vi "Update.vi"(8 "error in (no error)":errorcluster, 11 "Motions in":refnum<class "Motions.lvclass">) -> (0 "error out":errorcluster, 3 "Motions out":refnum<class "Motions.lvclass">)   [LabVIEW 2016, in "Hardware.lvlib" / "Motions.lvlib" / "Motions.lvclass"]
uses:
  <userlib>/Common Components/Hardware/Abstract System/Motions/Motions/Motions.lvclass
  <userlib>/Common Components/Hardware/Abstract System/Motions/Motions/Motions.lvclass/Motions.ctl
  <userlib>/Common Components/TriggerAction Q/TriggerAction Q/TriggerAction Q.lvclass/TriggerAction Q.ctl
  <userlib>/Common Components/TriggerAction Q/TriggerAction Q/Run (non-indexed).vi
  <userlib>/Common Components/Hardware/Motor/Motor/Motor.lvclass
  <userlib>/Common Components/TriggerAction Q/TriggerAction Q/TriggerAction Q.lvclass
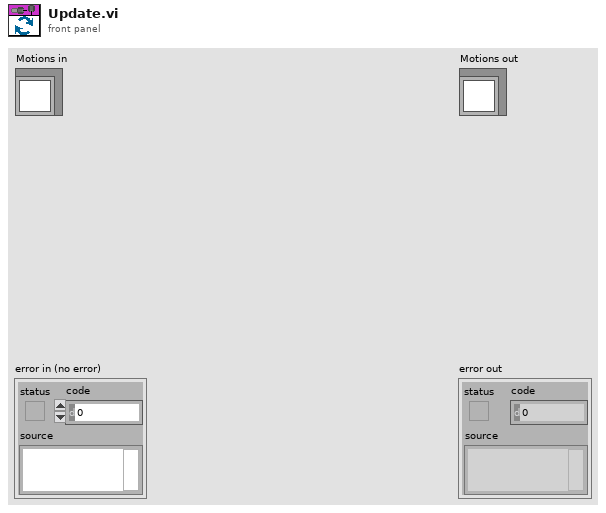
[diagram p1: front panel]
types:
  T1 = typedef "Hardware.lvlib/Motions.lvlib/Motions.lvclass/Motor States.ctl" = cluster{"Connected":bool, "Enabled":bool, "Moving Status":bool, "Soft Moving Status":bool, "Current Pos":dbl, "Target Pos":dbl, "Moving Dir (-1, 0, 1)":i32, "Error Status":bool, "Hard Limit+":bool, "Hard Limit-":bool, "Soft Limit+":bool, "Soft Limit-":bool, "History Dst Stack":refnum<queue>, "Motion Status":bool, "Motion TriggerAction Obj":refnum<class "TriggerAction Q.lvclass">, "Jogging":bool}
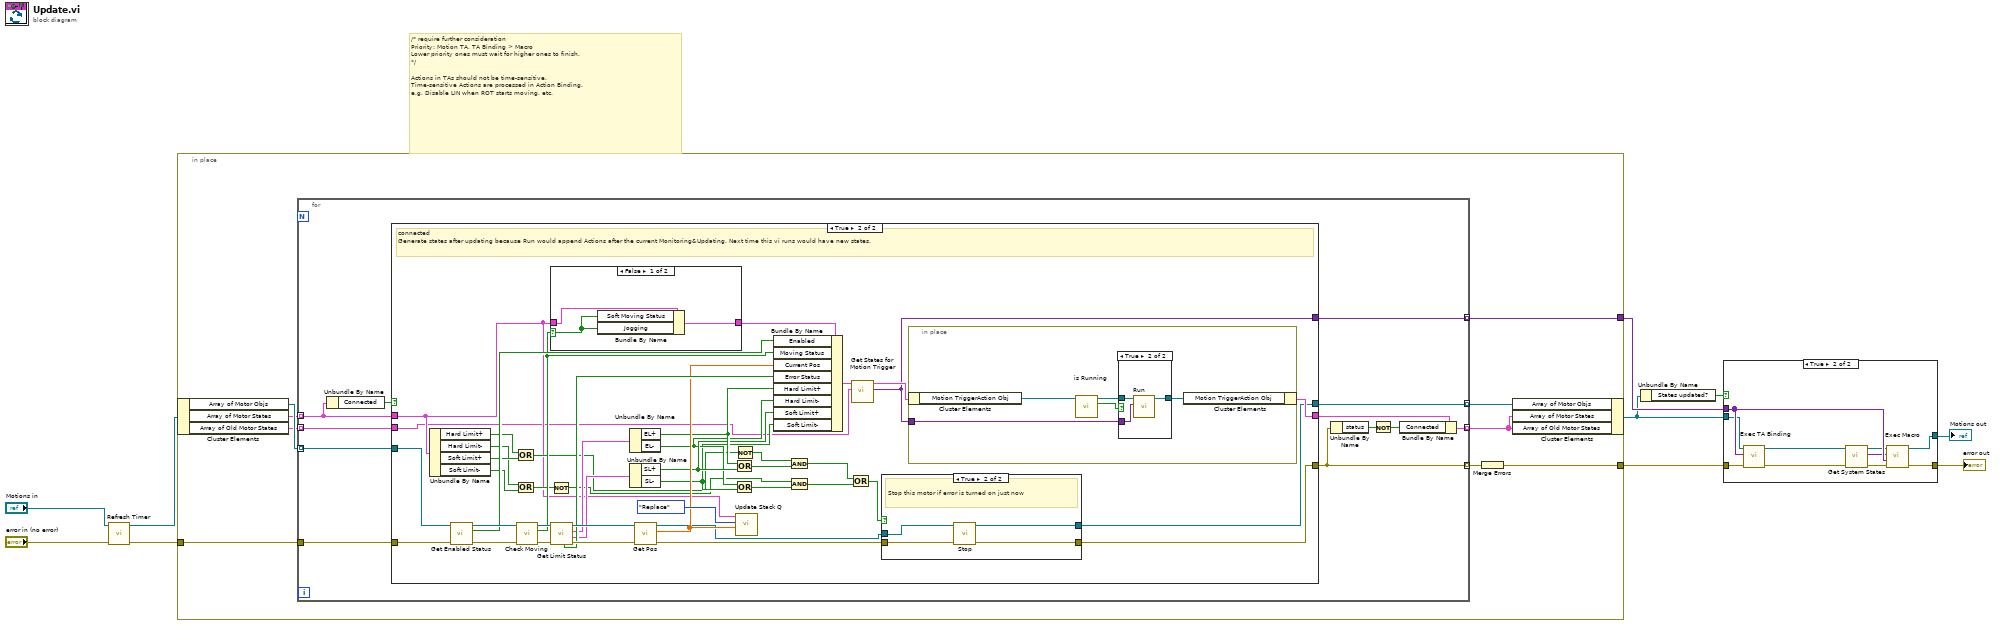
[diagram p0: block diagram]
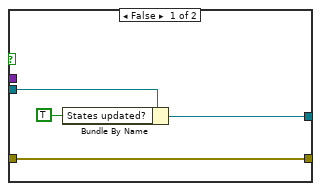
[diagram p2: hidden frame]
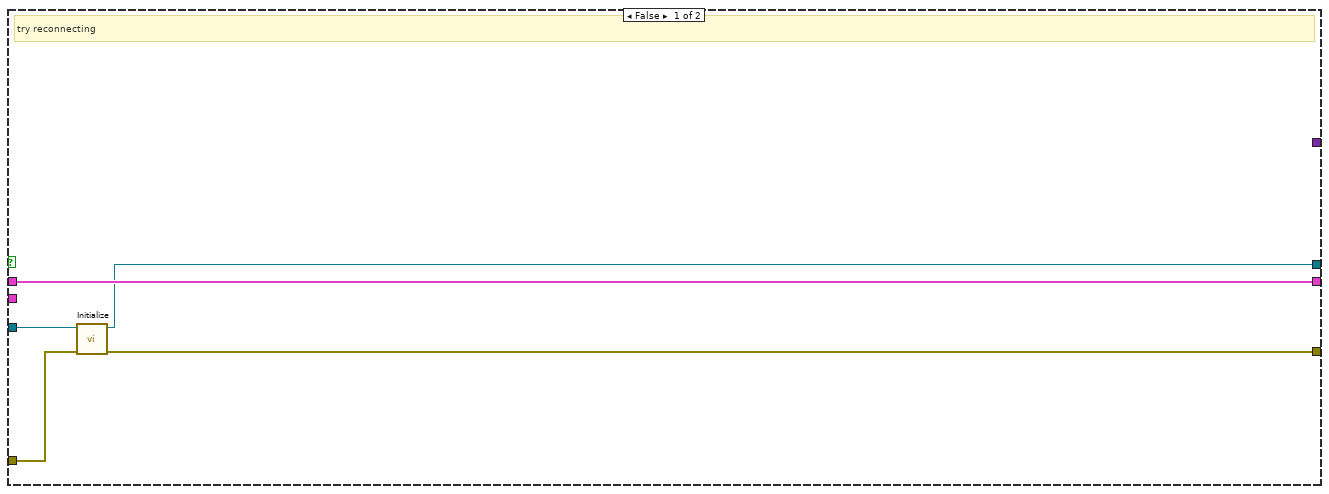
[diagram p3: hidden frame]
diagram:
  # "/* require further consideration\nPriority: Motion TA, TA Binding > Macro\nLower priority ones must wait for higher ones to finish.\n*/\n\nActions in TAs should not be time-sensitive.\nTime-sensitive Actions are processed in Action Binding.\ne.g. Disable LIN when ROT starts moving, etc."
  n1 = call <userlib>:"Refresh Timer.vi"("error in (no error)"="error in (no error)", "Motions in"="Motions in") -> ("error out"=w6:errorcluster, "Motions out"=w4:refnum<class "Motions.lvclass">)  [unwired: 8 in]
  n2 = in-place {
    in-place-border: w6 -> [w19]
    in-place-border: [w17] -> w9
    in-place-border: [w13] -> w3
    n3 = in-place-cluster #1(w4) -> ("Array of Motor Objs"=w16:refnum<class "Motor.lvclass">[], "Array of Motor States"=w15:T1[], "Array of Old Motor States"=w12:T1[])
    n4 = for {
      tunnel: w16 -> [w31] mode=indexing
      tunnel: w15 -> [w30] mode=indexing
      tunnel: [w26] -> w11 mode=indexing
      tunnel: w19 -> [w27]
      tunnel: [w25] -> w18 mode=indexing
      tunnel: [w22] -> w14 mode=indexing
      tunnel: [w21] -> w13 mode=indexing
      tunnel: w12 -> [w20] mode=indexing
      n5 = Unbundle By Name(w30) -> ("Connected"=w29:bool)
      n6 = case shown="True" w29 {
        tunnel: w31 -> [w35 w79]
        tunnel: w30 -> [w36 w38]
        tunnel: [w36 w63] -> w28
        tunnel: w27 -> [w34 w75]
        tunnel: [w33 w42] -> w25
        tunnel: [w32 w40] -> w22
        tunnel: [_ w59] -> w21
        tunnel: w20 -> [_ w37]
        frame False {
          # "try reconnecting"
          n7 = call-dynamic "Initialize.vi"("error in (no error)"=w34, "CCD in"=w35) -> ("error out"=w33:errorcluster, "CCD out"=w32:refnum<class "Motor.lvclass">)  [unwired: 8 in]
        }
        frame True {
          # "connected\nGenerate states after updating because Run would append Actions after the current Monitoring&Updating. Next time this vi runs would have new states."
          n8 = Unbundle By Name(w38) -> ("Hard Limit+"=w58:bool, "Hard Limit-"=w55:bool, "Soft Limit+"=w56:bool, "Soft Limit-"=w57:bool)
          n9 = call-dynamic "Get Enabled Status.vi"("error in (no error)"=w75, "Motor in"=w79) -> ("error out"=w74:errorcluster, "bENA"=w77:bool, "Motor out"=w78:refnum<class "Motor.lvclass">)  [unwired: 7 in]
          n10 = Or(x=w58, y=w56) -> (x .or. y?=w50:bool)
          n11 = Or(x=w55, y=w57) -> (x .or. y?=w47:bool)
          n12 = call-dynamic "Check Moving.vi"("error in (no error)"=w74, "Motor in"=w78) -> ("error out"=w73:errorcluster, "moving?"=w62:bool, "Motor out"=w70:refnum<class "Motor.lvclass">)  [unwired: 7 in]
          n13 = Not(x=w47) -> (.not. x?=w45:bool)
          n14 = case shown="False" w62 {
            selector: w62 -> [w95 _]
            tunnel: w38 -> [w97 w98]
            tunnel: [w96 w98] -> w76
            frame False {
              n15 = Bundle By Name(cluster=w97, "Soft Moving Status"=w95, "Jogging"=w95) -> (w96:T1)
            }
            frame True {
            }
          }
          n16 = call-dynamic "Get Limit Status.vi"("error in (no error)"=w73, "Motor in"=w70) -> ("error out"=w71:errorcluster, "Soft Limit status"=w66:cluster{"SL+":bool, "SL-":bool}, "EL status"=w67:cluster{"EL+":bool, "EL-":bool}, "Motor out"=w69:refnum<class "Motor.lvclass">, "ensemble Limit status"=w68:bool)  [unwired: 5 in]
          n17 = Unbundle By Name(w67) -> ("EL+"=w54:bool, "EL-"=w52:bool)
          n18 = Unbundle By Name(w66) -> ("SL+"=w53:bool, "SL-"=w51:bool)
          n19 = call <userlib>:"Get Pos.vi"("error in (no error)"=w71, "Motor in"=w69) -> ("error out"=w72:errorcluster, "Position in display unit (backend)"=w60:dbl, "Motor out"=w41:refnum<class "Motor.lvclass">)  [unwired: 6 in, 1 out]
          n20 = Or(x=w54, y=w53) -> (x .or. y?=w49:bool)
          n21 = Or(x=w52, y=w51) -> (x .or. y?=w46:bool)
          n22 = Not(x=w50) -> (.not. x?=w48:bool)
          n23 = call <userlib>:"Update Stack Q.vi"("Destination"=w60, "Mode"=enum16{"Add", "Replace"}."Replace", "Motor States"=w38) -> ()  [unwired: 9 in]
          n24 = Bundle By Name(cluster=w76, "Enabled"=w77, "Moving Status"=w62, "Current Pos"=w60, "Error Status"=w68, "Hard Limit+"=w54, "Hard Limit-"=w52, "Soft Limit+"=w53, "Soft Limit-"=w51) -> (w64:T1)
          n25 = And(x=w48, y=w49) -> (x .and. y?=w44:bool)
          n26 = And(x=w45, y=w46) -> (x .and. y?=w43:bool)
          n27 = Or(x=w44, y=w43) -> (x .or. y?=w39:bool)
          n28 = call <userlib>:"Get States for Motion Trigger.vi"("old Motor States in"=w37, "new Motor States in"=w64) -> ("States LUT (name -> boolean state)"=w59:variant, "new Motor States out"=w65:T1)  [unwired: 6 in, 2 out]
          n29 = case shown="True" w39 {
            tunnel: w72 -> [w80 w85]
            tunnel: [w80 w84] -> w42
            tunnel: w41 -> [w81 w83]
            tunnel: [w81 w82] -> w40
            frame False {
            }
            frame True {
              # "Stop this motor if error is turned on just now"
              n30 = call-dynamic "Stop.vi"("error in (no error)"=w85, "Motor in"=w83) -> ("error out"=w84:errorcluster, "Motor out"=w82:refnum<class "Motor.lvclass">)  [unwired: 8 in]
            }
          }
          n31 = in-place {
            in-place-border: w59 -> [w86]
            n32 = in-place-cluster #2(w65) -> ("Motion TriggerAction Obj"=w89:refnum<class "TriggerAction Q.lvclass">)
            n33 = call <userlib>:"is Running.vi"("TriggerAction in"=w89) -> ("Running?"=w87:bool, "TriggerAction out"=w90:refnum<class "TriggerAction Q.lvclass">)  [unwired: 9 in]
            n34 = case shown="True" w87 {
              tunnel: w90 -> [w91 w94]
              tunnel: [w91 w93] -> w88
              tunnel: w86 -> [_ w92]
              frame False {
              }
              frame True {
                n35 = call-poly <userlib>:"Run.vi"("States LUT (name -> boolean state)"=w92, "TriggerAction in"=w94) -> ("TriggerAction out"=w93:refnum<class "TriggerAction Q.lvclass">)  [unwired: 8 in, 1 out]
              }
            }
            n36 = in-place-cluster #2("Motion TriggerAction Obj"=w88) -> (w63:T1)
          }
        }
      }
      n37 = Unbundle By Name(w25) -> ("status"=w24:bool)
      n38 = Not(x=w24) -> (.not. x?=w23:bool)
      n39 = Bundle By Name(cluster=w28, "Connected"=w23) -> (w26:T1)
    }
    n40 = Merge Errors(w18) -> (w17:errorcluster)
    n41 = in-place-cluster #1("Array of Motor Objs"=w14, "Array of Motor States"=w11, "Array of Old Motor States"=w11) -> (w2:refnum<class "Motions.lvclass">)
  }
  n42 = Unbundle By Name(w2) -> ("States updated?"=w1:bool)
  n43 = case shown="True" w1 {
    tunnel: w9 -> [w101 w112]
    tunnel: [w101 w110] -> w8
    tunnel: [w100 w109] -> w7
    tunnel: w3 -> [_ w108]
    tunnel: w2 -> [w102 w103]
    frame False {
      n44 = Bundle By Name(cluster=w102, "States updated?"=TRUE ("States valid?")) -> (w100:refnum<class "Motions.lvclass">)
    }
    frame True {
      n45 = call <userlib>:"Exec TA Binding.vi"("error in (no error)"=w112, "Array of States LUT"=w108, "Motions in"=w103) -> ("error out"=w111:errorcluster, "Motions out"=w106:refnum<class "Motions.lvclass">)  [unwired: 7 in]
      n46 = call <userlib>:"Get System States.vi"("error in (no error)"=w111, "Motions in"=w106) -> ("error out"=w107:errorcluster, "States LUT (name -> boolean state)"=w104:variant, "Motions out"=w105:refnum<class "Motions.lvclass">)  [unwired: 6 in, 1 out]
      n47 = call <userlib>:"Exec Macro.vi"("error in (no error)"=w107, "Array of States LUT"=w108, "States LUT (name -> boolean state)"=w104, "Motions in"=w105) -> ("error out"=w110:errorcluster, "Motions out"=w109:refnum<class "Motions.lvclass">)  [unwired: 6 in]
    }
  }
  "error out" <- w8
  "Motions out" <- w7
